vi "PH_IEEE1394Camera.set Cam Attribute.vi"(0 "IMAQ1394 Session In":T3, 1 "Cam Attribute Name":string, 2 "Attribute Value Num":dbl, 3 "Attribute String / Command":string="CameraAttributes::Brightness::Value", 4 "Attribute Bool":bool, 5 "Cam Error in":errorcluster, 7 "Attribute Information Array":T2(array[cluster])) -> (14 "IMAQ1394 Session Out":T3, 15 "Attribute changed?":bool, 19 "Cam Error out":errorcluster)   [LabVIEW 2014, in "PH_IEEE1394Camera.lvlib"]
doc: "This VI sets the camera attribute."
uses:
  PH_IEEE1394Camera.lvlib
  <vilib>/userdefined/High Color/IMAQdx.ctl
  <vilib>/vision/driver/IMAQdx.llb/IMAQdx Attribute Type.ctl
  <resource>/objmgr/imaqdx.rc
  <vilib>/vision/driver/NI_Vision_Acquisition_Software.lvlib
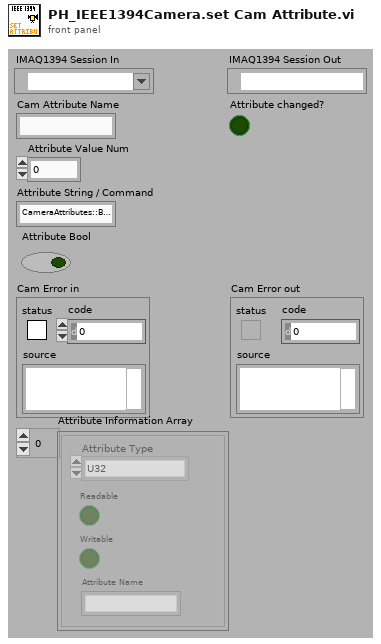
[diagram p1: front panel]
types:
  T1 = typedef "NI_Vision_Acquisition_Software.lvlib/IMAQdx Attribute Type.ctl" = enum32{"U32", "I64", "DBL", "String", "Enum", "Bool", "Command"}
  T2 = cluster{"Attribute Type":T1, "Readable":bool, "Writable":bool, "Attribute Name":string}[]
  T3 = typedef "IMAQdx.ctl" = refnum<k21>
  T4 = cluster{"Attribute Type":T1, "Readable":bool, "Writable":bool, "Attribute Name":string}
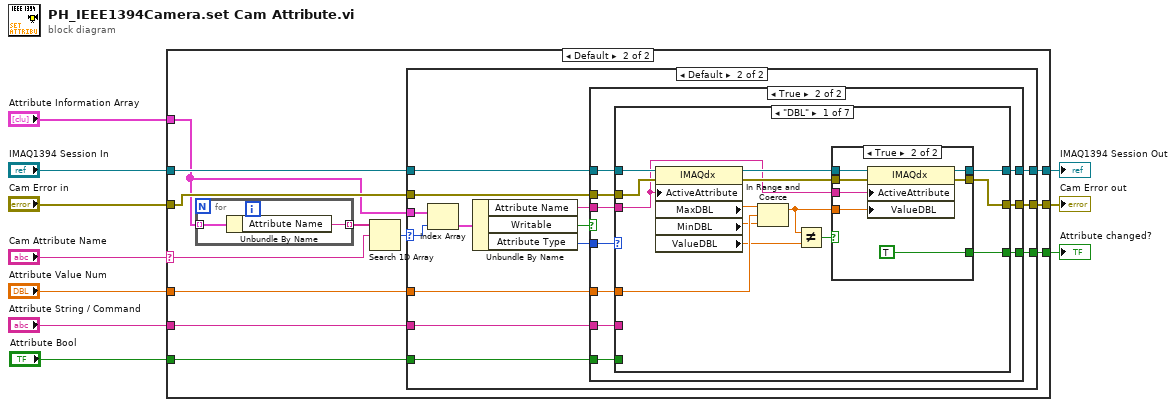
[diagram p0: block diagram]
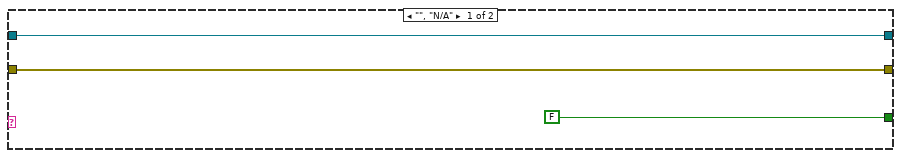
[diagram p2: hidden frame]
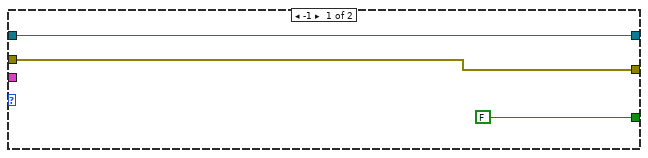
[diagram p3: hidden frame]
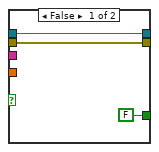
[diagram p5: hidden frame]
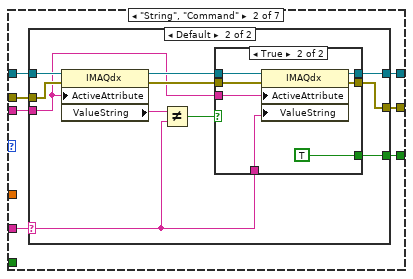
[diagram p6: hidden frame]
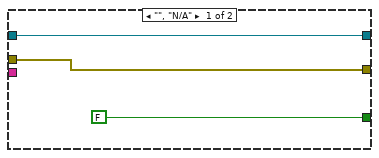
[diagram p7: hidden frame]
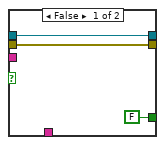
[diagram p8: hidden frame]
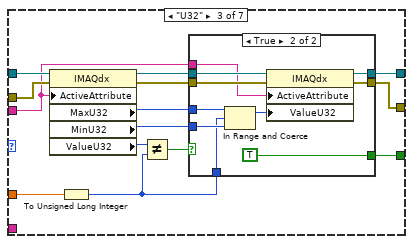
[diagram p9: hidden frame]
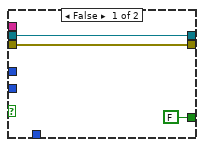
[diagram p10: hidden frame]
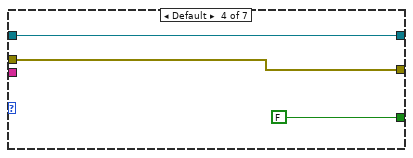
[diagram p11: hidden frame]
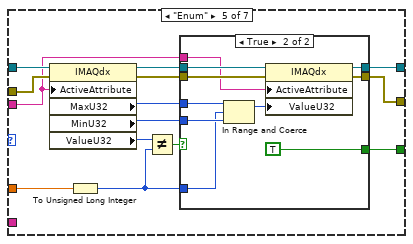
[diagram p12: hidden frame]
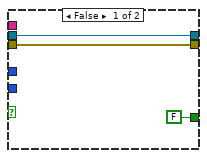
[diagram p13: hidden frame]
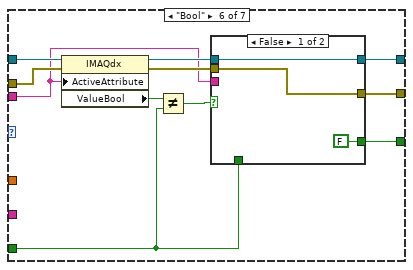
[diagram p14: hidden frame]
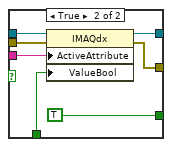
[diagram p15: hidden frame]
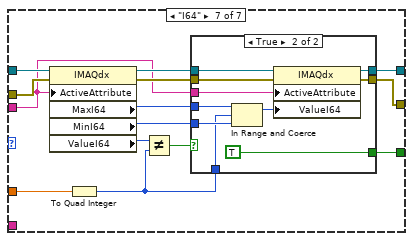
[diagram p16: hidden frame]
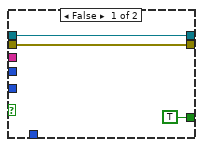
[diagram p17: hidden frame]
diagram:
  n1 = case shown="Default" "Cam Attribute Name" {
    selector: "Cam Attribute Name" -> [_ w18]
    tunnel: [w13 w25] -> w10
    tunnel: [w12 w24] -> w9
    tunnel: "Cam Error in" -> [w12 w23]
    tunnel: "IMAQ1394 Session In" -> [w13 w17]
    tunnel: [FALSE w22] -> w6
    tunnel: "Attribute Value Num" -> [_ w21]
    tunnel: "Attribute String / Command" -> [_ w20]
    tunnel: "Attribute Bool" -> [_ w19]
    tunnel: "Attribute Information Array" -> [_ w16]
    frame "", "N/A" {
    }
    frame Default {
      n2 = for {
        tunnel: w16 -> [w217] mode=indexing
        tunnel: [w216] -> w15 mode=indexing
        n3 = Unbundle By Name(w217) -> ("Attribute Name"=w216:string)
      }
      n4 = Search 1D Array(1D array=w15, element=w18) -> (index of element=w14:i32)  [unwired: 1 in]
      n5 = case shown="Default" w14 {
        selector: w14 -> [_ w36]
        tunnel: [w27 w42] -> w25
        tunnel: w23 -> [w28 w41]
        tunnel: [w28 w40] -> w24
        tunnel: w17 -> [w27 w39]
        tunnel: w16 -> [_ w38]
        tunnel: [FALSE w33] -> w22
        tunnel: w21 -> [_ w31]
        tunnel: w20 -> [_ w30]
        tunnel: w19 -> [_ w29]
        frame -1 {
        }
        frame Default {
          n6 = Index Array(array=w38, index=w36) -> (element=w37:T4)
          n7 = Unbundle By Name(w37) -> ("Attribute Name"=w35:string, "Writable"=w34:bool, "Attribute Type"=w32:T1)
          n8 = case shown="True" w34 {
            selector: w34 -> [w43 _]
            tunnel: [w45 w55] -> w42
            tunnel: w41 -> [w44 w54]
            tunnel: [w44 w53] -> w40
            tunnel: w39 -> [w45 w52]
            tunnel: w35 -> [_ w51]
            tunnel: [w43 w48] -> w33
            tunnel: w32 -> [_ w50]
            tunnel: w31 -> [_ w49]
            tunnel: w30 -> [_ w47]
            tunnel: w29 -> [_ w46]
            frame False {
            }
            frame True {
              n9 = case shown="\"DBL\"" w50 {
                tunnel: [w66 w84 w119 w139 w149 w178 w197] -> w55
                tunnel: w54 -> [w69 w86 w124 w138 w154 w173 w202]
                tunnel: [w64 w83 w117 w138 w147 w177 w195] -> w53
                tunnel: w52 -> [w68 w85 w123 w139 w153 w175 w201]
                tunnel: w51 -> [w63 w82 w116 _ w146 w171 w194]
                tunnel: w49 -> [w60 _ w115 _ w145 _ w193]
                tunnel: [w62 w81 w114 FALSE w144 w176 w192] -> w48
                tunnel: w47 -> [_ w80 _ _ _ _ _]
                tunnel: w46 -> [_ _ _ _ _ w169 _]
                frame "DBL" {
                  n10 = property class="IMAQdx"(reference=w68, error in=w69, "ActiveAttribute"=w63) -> (reference out=w67:T3, error out=w65:errorcluster, "MaxDBL"=w59:dbl, "MinDBL"=w58:dbl, "ValueDBL"=w56:dbl)
                  n11 = In Range and Coerce(upper limit=w59, x=w60, lower limit=w58) -> (coerced(x)=w57:dbl)  [unwired: 1 out]
                  n12 = Not Equal?(x=w57, y=w56) -> (x != y?=w61:bool)
                  n13 = case shown="True" w61 {
                    tunnel: w67 -> [w72 w79]
                    tunnel: [w72 w78] -> w66
                    tunnel: w65 -> [w71 w77]
                    tunnel: [w71 w76] -> w64
                    tunnel: w63 -> [_ w75]
                    tunnel: [FALSE TRUE] -> w62
                    tunnel: w57 -> [_ w73]
                    frame False {
                    }
                    frame True {
                      n14 = property class="IMAQdx"(reference=w79, error in=w77, "ActiveAttribute"=w75, "ValueDBL"=w73) -> (reference out=w78:T3, error out=w76:errorcluster)
                    }
                  }
                }
                frame "String", "Command" {
                  n15 = case shown="Default" w80 {
                    selector: w80 -> [_ w92]
                    tunnel: w86 -> [w88 w95]
                    tunnel: w85 -> [w89 w97]
                    tunnel: [w89 w100] -> w84
                    tunnel: [w88 w99] -> w83
                    tunnel: w82 -> [_ w90]
                    tunnel: [FALSE w98] -> w81
                    frame "", "N/A" {
                    }
                    frame Default {
                      n16 = property class="IMAQdx"(reference=w97, error in=w95, "ActiveAttribute"=w90) -> (reference out=w96:T3, error out=w94:errorcluster, "ValueString"=w93:string)
                      n17 = Not Equal?(x=w93, y=w92) -> (x != y?=w91:bool)
                      n18 = case shown="True" w91 {
                        tunnel: [w103 w110] -> w100
                        tunnel: [w102 w109] -> w99
                        tunnel: w92 -> [_ w108]
                        tunnel: [FALSE TRUE] -> w98
                        tunnel: w96 -> [w103 w106]
                        tunnel: w94 -> [w102 w105]
                        tunnel: w90 -> [_ w104]
                        frame False {
                        }
                        frame True {
                          n19 = property class="IMAQdx"(reference=w106, error in=w105, "ActiveAttribute"=w104, "ValueString"=w108) -> (reference out=w110:T3, error out=w109:errorcluster)
                        }
                      }
                    }
                  }
                }
                frame "U32" {
                  n20 = property class="IMAQdx"(reference=w123, error in=w124, "ActiveAttribute"=w116) -> (reference out=w120:T3, error out=w118:errorcluster, "MaxU32"=w122:u32, "MinU32"=w121:u32, "ValueU32"=w113:u32)
                  n21 = To Unsigned Long Integer(number=w115) -> (unsigned 32bit integer=w111:u32)
                  n22 = Not Equal?(x=w113, y=w111) -> (x != y?=w112:bool)
                  n23 = case shown="True" w112 {
                    tunnel: w122 -> [_ w137]
                    tunnel: w121 -> [_ w136]
                    tunnel: w120 -> [w127 w135]
                    tunnel: [w127 w134] -> w119
                    tunnel: w118 -> [w126 w133]
                    tunnel: [w126 w132] -> w117
                    tunnel: w116 -> [_ w131]
                    tunnel: w111 -> [_ w130]
                    tunnel: [FALSE TRUE] -> w114
                    frame False {
                    }
                    frame True {
                      n24 = In Range and Coerce(upper limit=w137, x=w130, lower limit=w136) -> (coerced(x)=w129:u32)  [unwired: 1 out]
                      n25 = property class="IMAQdx"(reference=w135, error in=w133, "ActiveAttribute"=w131, "ValueU32"=w129) -> (reference out=w134:T3, error out=w132:errorcluster)
                    }
                  }
                }
                frame Default {
                }
                frame "Enum" {
                  n26 = property class="IMAQdx"(reference=w153, error in=w154, "ActiveAttribute"=w146) -> (reference out=w150:T3, error out=w148:errorcluster, "MaxU32"=w152:u32, "MinU32"=w151:u32, "ValueU32"=w143:u32)
                  n27 = To Unsigned Long Integer(number=w145) -> (unsigned 32bit integer=w141:u32)
                  n28 = Not Equal?(x=w143, y=w141) -> (x != y?=w142:bool)
                  n29 = case shown="True" w142 {
                    tunnel: w152 -> [_ w167]
                    tunnel: w151 -> [_ w166]
                    tunnel: w150 -> [w157 w165]
                    tunnel: [w157 w164] -> w149
                    tunnel: w148 -> [w156 w163]
                    tunnel: [w156 w162] -> w147
                    tunnel: w146 -> [_ w161]
                    tunnel: w141 -> [_ w160]
                    tunnel: [FALSE TRUE] -> w144
                    frame False {
                    }
                    frame True {
                      n30 = In Range and Coerce(upper limit=w167, x=w160, lower limit=w166) -> (coerced(x)=w159:u32)  [unwired: 1 out]
                      n31 = property class="IMAQdx"(reference=w165, error in=w163, "ActiveAttribute"=w161, "ValueU32"=w159) -> (reference out=w164:T3, error out=w162:errorcluster)
                    }
                  }
                }
                frame "Bool" {
                  n32 = property class="IMAQdx"(reference=w175, error in=w173, "ActiveAttribute"=w171) -> (reference out=w174:T3, error out=w172:errorcluster, "ValueBool"=w170:bool)
                  n33 = Not Equal?(x=w170, y=w169) -> (x != y?=w168:bool)
                  n34 = case shown="False" w168 {
                    tunnel: [w180 w188] -> w178
                    tunnel: [w181 w187] -> w177
                    tunnel: w169 -> [_ w186]
                    tunnel: [FALSE TRUE] -> w176
                    tunnel: w174 -> [w180 w184]
                    tunnel: w172 -> [w181 w183]
                    tunnel: w171 -> [_ w182]
                    frame False {
                    }
                    frame True {
                      n35 = property class="IMAQdx"(reference=w184, error in=w183, "ActiveAttribute"=w182, "ValueBool"=w186) -> (reference out=w188:T3, error out=w187:errorcluster)
                    }
                  }
                }
                frame "I64" {
                  n36 = property class="IMAQdx"(reference=w201, error in=w202, "ActiveAttribute"=w194) -> (reference out=w198:T3, error out=w196:errorcluster, "MaxI64"=w200:i64, "MinI64"=w199:i64, "ValueI64"=w191:i64)
                  n37 = To Quad Integer(1:w193) -> (0:w190:i64)
                  n38 = Not Equal?(x=w191, y=w190) -> (x != y?=w189:bool)
                  n39 = case shown="True" w189 {
                    tunnel: w200 -> [_ w215]
                    tunnel: w199 -> [_ w214]
                    tunnel: w198 -> [w205 w213]
                    tunnel: [w205 w212] -> w197
                    tunnel: w196 -> [w204 w211]
                    tunnel: [w204 w210] -> w195
                    tunnel: w194 -> [_ w209]
                    tunnel: w190 -> [_ w208]
                    tunnel: [TRUE TRUE] -> w192
                    frame False {
                    }
                    frame True {
                      n40 = In Range and Coerce(upper limit=w215, x=w208, lower limit=w214) -> (coerced(x)=w207:i64)  [unwired: 1 out]
                      n41 = property class="IMAQdx"(reference=w213, error in=w211, "ActiveAttribute"=w209, "ValueI64"=w207) -> (reference out=w212:T3, error out=w210:errorcluster)
                    }
                  }
                }
              }
            }
          }
        }
      }
    }
  }
  "Cam Error out" <- w9
  "Attribute changed?" <- w6
  "IMAQ1394 Session Out" <- w10
